vi "4Pi Dual DM - Pixel Scan Engine.vi"(0 "Pixel Scan Parameters In":T1={"Scan Start Pixel"=1, "Scan End Pixel"=1, "Pixel Start Value (-1 to 1)"=-0.5, "Pixel End Value (-1 to 1)"=0.5, "Number of Steps"=0.1}, 2 "Action":T2(ring), 11 "Initial Pixel Values (-1 to 1)":dbl[](array[numeric])) -> ()   [LabVIEW 2014]
uses:
  Controls/Pixel Scan Parameters.ctl
  Controls/Standard_Counter_Action.ctl
  Controls/Standard Action.ctl
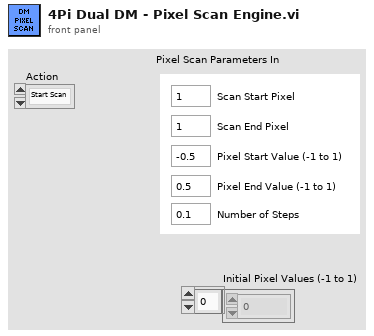
[diagram p1: front panel]
types:
  T1 = typedef "Pixel Scan Parameters.ctl" = cluster{"Scan Start Pixel":i32, "Scan End Pixel":i32, "Pixel Start Value (-1 to 1)":dbl, "Pixel End Value (-1 to 1)":dbl, "Number of Steps":dbl}
  T2 = enum16{"Start Scan", "Reset Counter", "Write DM", "Get Image", "Update Count", "Exit"}
  T3 = typedef "Standard_Counter_Action.ctl" = enum16{"Initialize", "Update Count", "Get Count"}
  T4 = typedef "Standard Action.ctl" = enum16{"Read", "Write"}
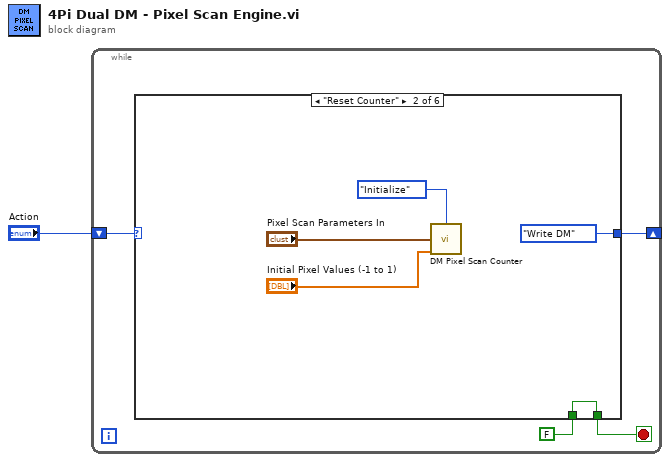
[diagram p0: block diagram]
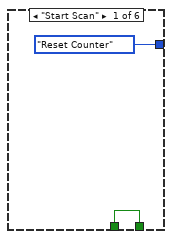
[diagram p2: hidden frame]
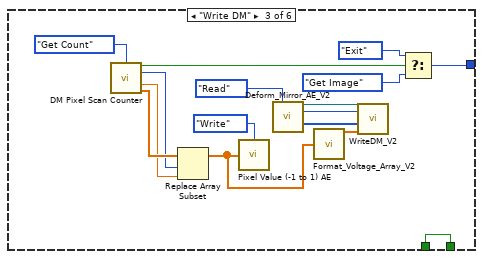
[diagram p3: hidden frame]
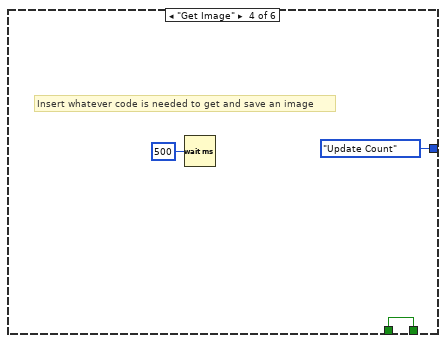
[diagram p4: hidden frame]
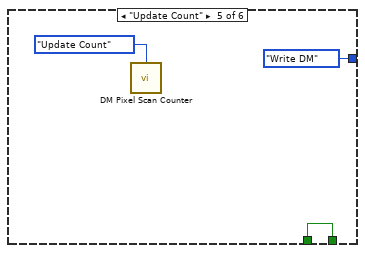
[diagram p5: hidden frame]
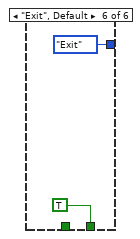
[diagram p6: hidden frame]
diagram:
  n1 = while {
    shift-right: [w2] -> _
    shift-left: "Action" -> [w5]
    stop <- w4 stop-if-true
    n2 = case shown="\"Reset Counter\"" w5 {
      tunnel: [w7 w9 w17 w31 w33 TRUE] -> w4
      tunnel: FALSE -> [w7 w9 w17 w31 w33 _]
      tunnel: [T2."Reset Counter" ("Action") T2."Write DM" ("Action") w18 T2."Update Count" ("Action") T2."Write DM" ("Action") T2."Exit" ("Action")] -> w2
      frame "Start Scan" {
      }
      frame "Reset Counter" {
        n3 = call "DM Pixel Scan Counter.vi"("Action"=Standard_Counter_Action."Initialize", "Pixel Scan Parameters In"="Pixel Scan Parameters In", "Initial Pixel Values (-1 to 1)"="Initial Pixel Values (-1 to 1)") -> ()  [unwired: 9 in, 4 out]
      }
      frame "Write DM" {
        n4 = call "DM Pixel Scan Counter.vi"("Action"=Standard_Counter_Action."Get Count") -> ("Scan Done"=w19:bool, "DM Pixel"=w25:i32, "Normalized DM Pixel Value"=w23:dbl, "Initial Pixel Values OUT"=w26:dbl[])  [unwired: 11 in]
        n5 = Replace Array Subset(array=w26, new element=w23, index=w25) -> (w24:dbl[])
        n6 = call "Pixel Value (-1 to 1) AE.vi"("Action"=Standard_Action."Write", "Pixel Value (-1 to 1)"=w24) -> ()  [unwired: 13 in, 1 out]
        n7 = call "Deform_Mirror_AE_V2.vi"("Action"=Standard_Action."Read") -> ("Refnum Out"=w20:refnum<k7>, "IDs Out"=w21:i32, "Multi Map Data Out"=w22:i32[])  [unwired: 10 in, 2 out]
        n8 = call "Format_Voltage_Array_V2.vi"("Pixel Level (-1 to 1)"=w24) -> ("Voltage Array (Volts)"=w16:dbl[])  [unwired: 13 in, 1 out]
        n9 = call "WriteDM_V2.vi"("reference in"=w20, "nDevId"=w21, "MultiDM  Mapping"=w22, "Voltage Array in"=w16) -> ()  [unwired: 2 in, 2 out]
        n10 = Select(t=T2."Exit" ("Action"), s=w19, f=T2."Get Image" ("Action")) -> (s? t:f=w18:T2)
      }
      frame "Get Image" {
        # "Insert whatever code is needed to get and save an image"
        n11 = Wait (ms)(milliseconds to wait=u32 500) -> ()  [unwired: 1 out]
      }
      frame "Update Count" {
        n12 = call "DM Pixel Scan Counter.vi"("Action"=Standard_Counter_Action."Update Count") -> ()  [unwired: 11 in, 4 out]
      }
      frame "Exit", Default {
      }
    }
  }
